vi "getOdoConf.vi"(8 "error in (no error)":errorcluster, 11 "pHandle":u32) -> (0 "error out":errorcluster, 1 "return type":i32, 3 "axisStr":string)   [LabVIEW 2011, in "sbgLabView.lvlib"]
uses:
  sbgLabView.lvlib
  sbgMatLab.dll
panel:
  out "gpsGainCorrection":bool
  out "GainError":u8
  out "pulsesPerMeter":sgl
  in  "channel":u8
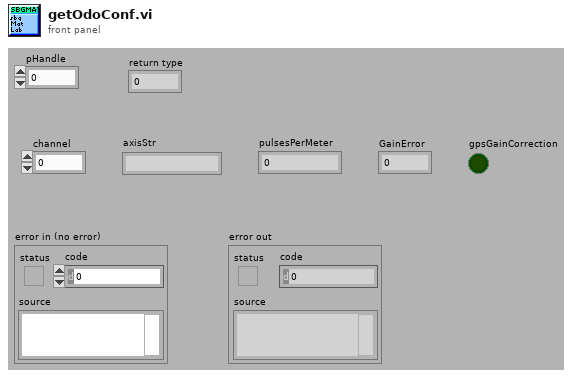
[diagram p1: front panel]
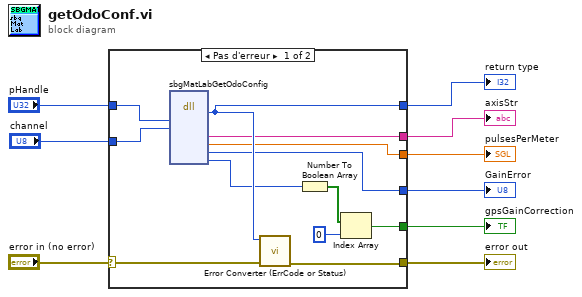
[diagram p0: block diagram]
diagram:
  n1 = case shown="Pas d'erreur" "error in (no error)" {
    selector: "error in (no error)" -> [w18 w22]
    tunnel: [w17 w22] -> w8
    tunnel: [w21 _] -> w7
    tunnel: "pHandle" -> [w20 _]
    tunnel: [w19 _] -> w5
    tunnel: [w14 _] -> w4
    tunnel: [w12 _] -> w3
    tunnel: [w11 _] -> w2
    tunnel: "channel" -> [w10 _]
    frame No Error {
      n2 = dll-call lib="C:/SBG-Systems/remote/projects/software/projects/labviewExample/sbgLabView/sbgMatLab.*" fn="sbgMatLabGetOdoConfig" ("sbgMatLab.dll:sbgMatLabGetGpsOptions")("pHandle"=w20, "channel"=w10) -> ("type de retour"=w21:i32, "axisStr"=w19:string, "pPulsesPerMeter"=w11:sgl, "pGainError"=w12:u8, "pGpsGainCorrection"=w13:u8)  [unwired: 9 in, 2 out]
      n3 = call "Error Converter (ErrCode or Status).vi"("error in (no error)"=w18, "error code"=w21) -> ("error out"=w17:errorcluster)  [unwired: 9 in]
      n4 = Number To Boolean Array(number=w13) -> (Boolean array=w16:bool[])
      n5 = Index Array(array=w16, index=0) -> (element=w14:bool)
    }
    frame Error {
    }
  }
  "return type" <- w7
  "axisStr" <- w5
  "error out" <- w8
  "pulsesPerMeter" <- w2
  "GainError" <- w3
  "gpsGainCorrection" <- w4
